vi "Read Current State Status.vi"(8 "error in (no error)":errorcluster, 11 "Command States in":refnum<class "Command States.lvclass">) -> (0 "error out":errorcluster, 2 "State Status":T1, 3 "Command States out":refnum<class "Command States.lvclass">)   [LabVIEW 2013, in "Command Actor.lvlib" / "Command States.lvclass"]
uses:
  Command States.lvclass
  Command/State Status.ctl
  Command States.lvclass/Command States.ctl
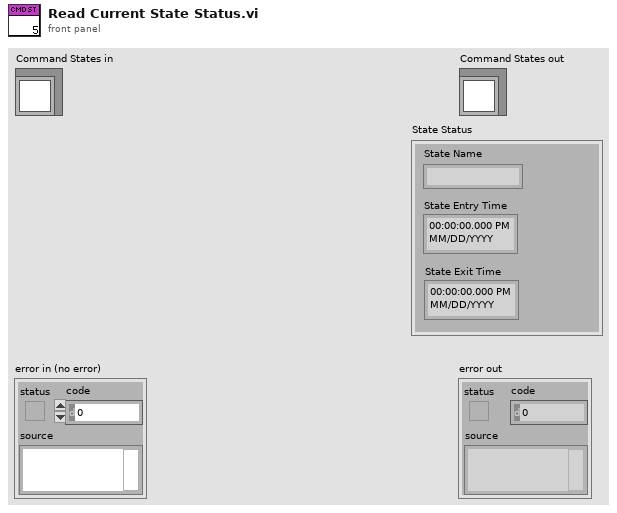
[diagram p1: front panel]
types:
  T1 = typedef "Command Actor.lvlib/Command States.lvclass/State Status.ctl" = cluster{"State Name":string, "State Entry Time":timestamp, "State Exit Time":timestamp}
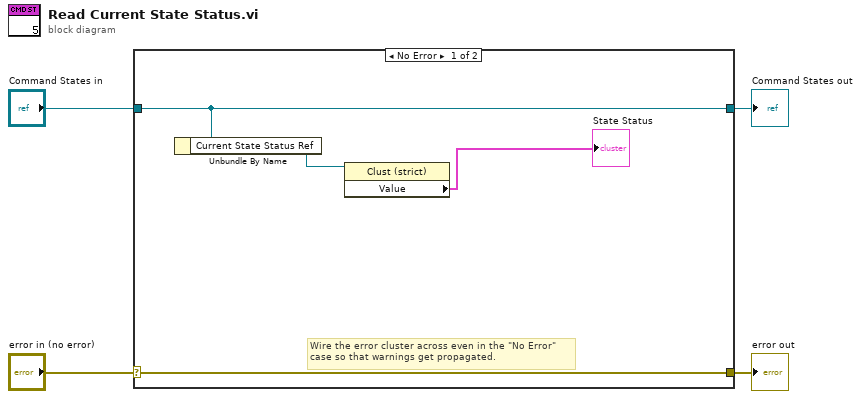
[diagram p0: block diagram]
diagram:
  n1 = case shown="No Error" "error in (no error)" {
    selector: "error in (no error)" -> [w8 w10]
    tunnel: [w8 w10] -> w3
    tunnel: [w7 w9] -> w1
    tunnel: "Command States in" -> [w7 w9]
    frame No Error {
      # "Wire the error cluster across even in the \"No Error\"\ncase so that warnings get propagated."
      n2 = Unbundle By Name(w7) -> ("Current State Status Ref"=w6:refnum<vi>)
      n3 = property class="Clust (strict)"(reference=w6) -> ("Value"=→"State Status":T1)  [unwired: 1 in, 2 out]
    }
    frame Error {
    }
  }
  "error out" <- w3
  "Command States out" <- w1
